vi "Remove Outliers.vi"(1 "Distances (ft)":dbl[](array[numeric])) -> (0 "Mean Distance":dbl)   [LabVIEW 2014]
uses:
  <vilib>/gmath/NI_Gmath.lvlib
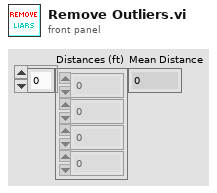
[diagram p1: front panel]
types:
  T1 = enum16{"arithmetic", "geometric", "harmonic", "trimmed", "median"}
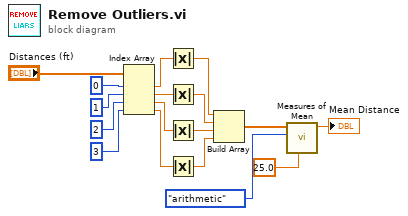
[diagram p0: block diagram]
diagram:
  n1 = Index Array(array="Distances (ft)", index #1=0 ("index"), index #2=1 ("index"), index #3=2 ("index"), index #4=3 ("index")) -> (element #1=w3:dbl, element #2=w1:dbl, element #3=w7:dbl, element #4=w6:dbl)
  n2 = Absolute Value(x=w3) -> (abs(x)=w4:dbl)
  n3 = Absolute Value(x=w1) -> (abs(x)=w2:dbl)
  n4 = Absolute Value(x=w7) -> (abs(x)=w8:dbl)
  n5 = Absolute Value(x=w6) -> (abs(x)=w5:dbl)
  n6 = Build Array(w4, w2, w8, w5) -> (w9:dbl[])
  n7 = call <vilib>:"Measures of Mean.vi"("percent (trim)"=25.0, "type"=T1."arithmetic", "x array"=w9) -> ("mean value"=→"Mean Distance":dbl)  [unwired: 7 in, 1 out]
